vi "Agilent DMM Release.vi"(7 "Agilent DMM":T1, 8 "error in (no error)":errorcluster, 11 "VISA Resource Name":refnum<visa-resource-name>) -> (0 "error out":errorcluster {"code" format="%.0x"})   [LabVIEW 2011]
uses:
  TypeDefs/Agilent DMM Instrument Info.ctl
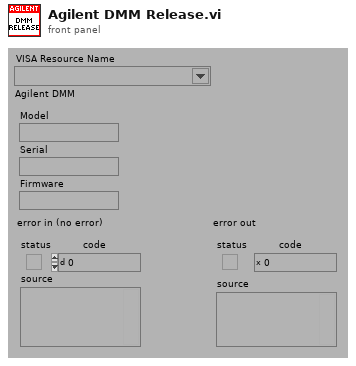
[diagram p1: front panel]
types:
  T1 = typedef "Agilent DMM Instrument Info.ctl" = cluster{"Model":string, "Serial":string, "Firmware":string}
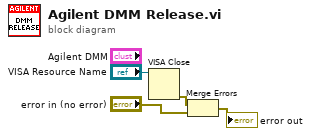
[diagram p0: block diagram]
diagram:
  n1 = VISA Close(VISA resource name="VISA Resource Name") -> (error out=w2:errorcluster)  [unwired: 1 in]
  n2 = Merge Errors(w2, "error in (no error)") -> (→"error out":errorcluster)
